vi "13.vi"() -> ()   [LabVIEW 2021]
panel:
  out "Numeric":u64
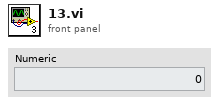
[diagram p1: front panel]
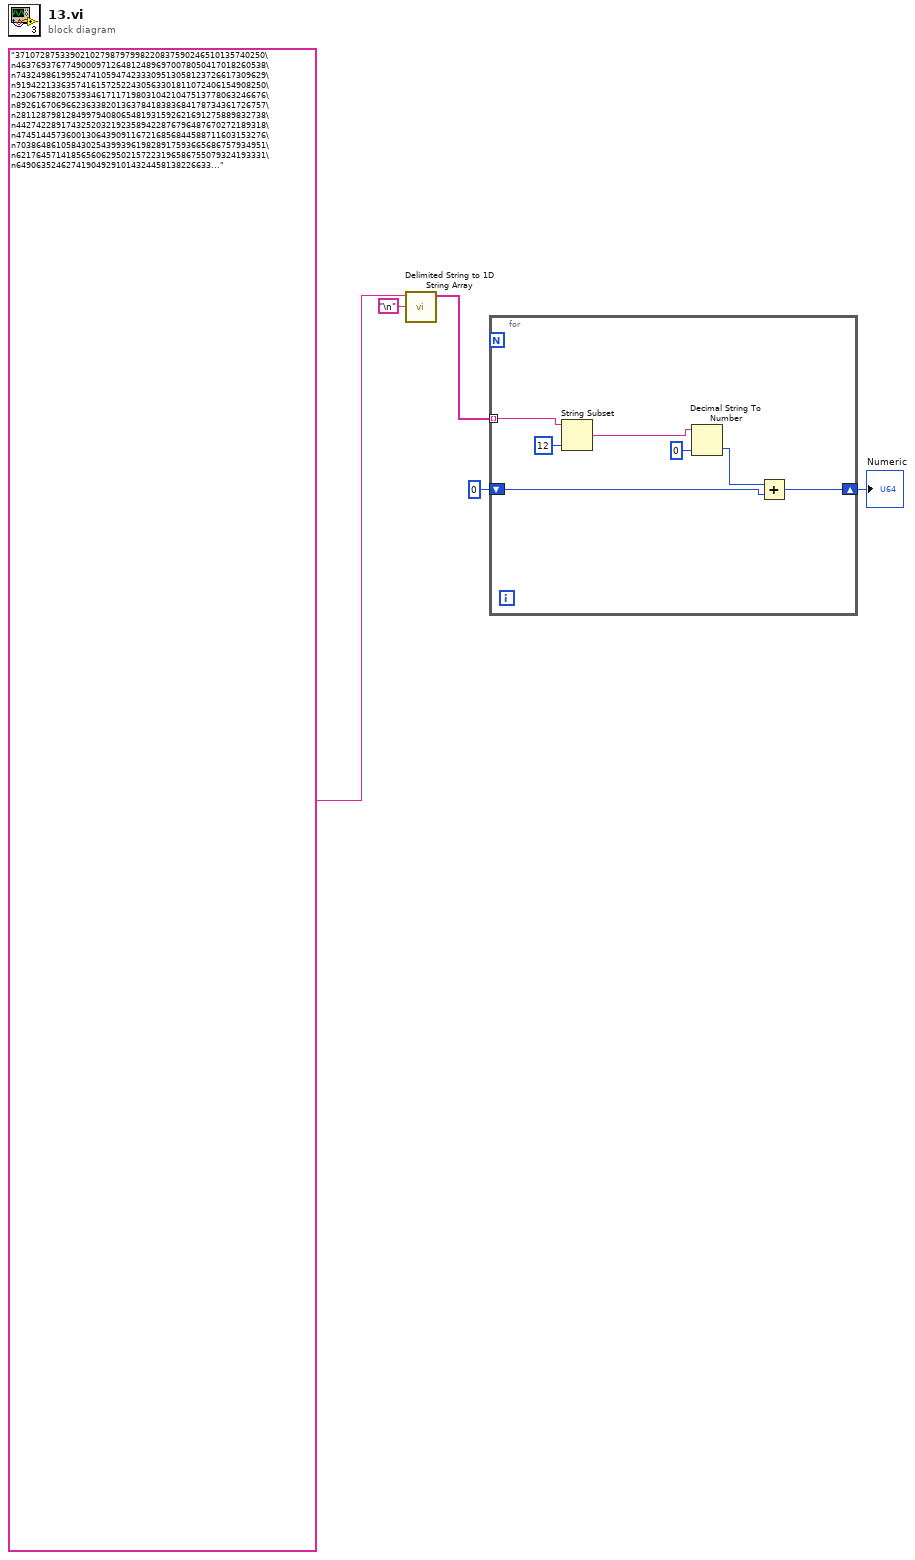
[diagram p0: block diagram]
diagram:
  n1 = call <vilib>:"Delimited String to 1D String Array.vi"("delimiter"="\n", "delimited string"="37107287533902102798797998220837590246510135740250\n46376937677490009712648124896970078050417018260538\n74324986199524741059474233309513058123726617309629\n91942213363574161572522430563301811072406154908250\n23067588207539346171171980310421047513778063246676\n89261670696623633820136378418383684178734361726757\n28112879812849979408065481931592621691275889832738\n44274228917432520321923589422876796487670272189318\n47451445736001306439091167216856844588711603153276\n70386486105843025439939619828917593665686757934951\n62176457141856560629502157223196586755079324193331\n649063524627419049291014324458138226633...") -> ("string array"=w3:string[])  [unwired: 9 in]
  n2 = for {
    tunnel: w3 -> [w12] mode=indexing
    shift-right: [w6] -> w1
    shift-left: u64 0 -> [w7]
    n3 = String Subset(string=w12, length (rest)=12 ("length (rest)")) -> (substring=w10:string)  [unwired: 1 in]
    n4 = Decimal String To Number(string=w10, default (0L)=u64 0 ("default (0 I32)")) -> (number=w8:u64)  [unwired: 1 in, 1 out]
    n5 = Add(x=w8, y=w7) -> (x+y=w6:u64)
  }
  "Numeric" <- w1
